vi "_Record Expt Header.vi"(1 "Expt/Cycle#":u16, 2 "Run Time (mS)":u32) -> ()   [LabVIEW 2012]
uses:
  <vilib>/rvi/DataTransferAndStorage/Container/XNode/niFpgaContainer.xnode
  <vilib>/rvi/interface/RandomDataEmulation/nirviRandomDataFpgaReadWriteTemplate.vi
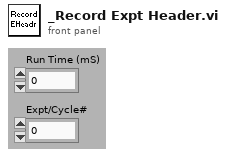
[diagram p1: front panel]
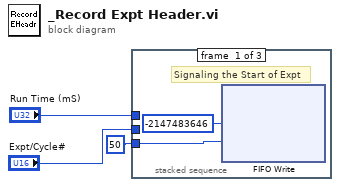
[diagram p0: block diagram]
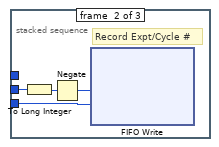
[diagram p2: hidden frame]
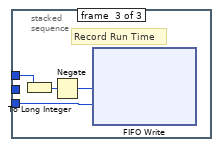
[diagram p3: hidden frame]
diagram:
  n1 = stacked-sequence {
    tunnel: "Expt/Cycle#" -> [_ w6 _]
    tunnel: u8 50 ("Timeout (-1 for no timeout)") -> [w4 w7 w11]
    tunnel: "Run Time (mS)" -> [_ _ w12]
    frame #0 {
      # "Signaling the Start of Expt"
      n2 = xnode ("FIFO Write")("Element"=-2147483646, "Timeout"=w4) -> ()  [unwired: 1 in, 2 out]
    }
    frame #1 {
      # "Record Expt/Cycle #"
      n3 = To Long Integer(number=w6) -> (32bit integer=w8:i32)
      n4 = Negate(x=w8) -> (-x=w9:i32)
      n5 = xnode ("FIFO Write")("Element"=w9, "Timeout"=w7) -> ()  [unwired: 1 in, 2 out]
    }
    frame #2 {
      # "Record Run Time"
      n6 = To Long Integer(number=w12) -> (32bit integer=w13:i32)
      n7 = Negate(x=w13) -> (-x=w10:i32)
      n8 = xnode ("FIFO Write")("Element"=w10, "Timeout"=w11) -> ()  [unwired: 1 in, 2 out]
    }
  }
